vi "Rayon max.vi"(8 "error in (no error)":T1 caption="entrée d'erreur (pas d'erreur)", 10 "Capteur 3 ou 4":dbl[](array[numeric]), 11 "Capteur 2":dbl[](array[numeric])) -> (0 "error out":T1 caption="sortie d'erreur", 3 "Rayon max":dbl)   [LabVIEW 2018]
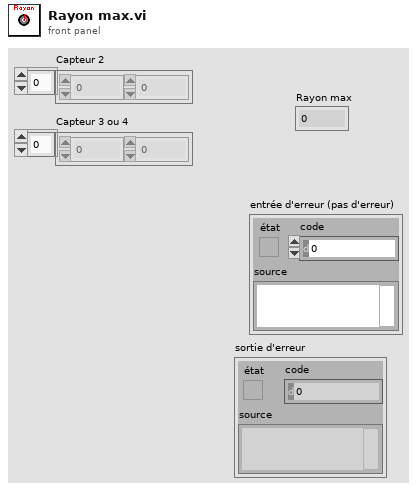
[diagram p1: front panel]
types:
  T1 = cluster{"état":bool, "code":i32, "source":string}
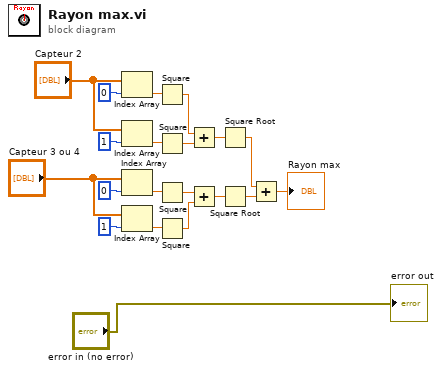
[diagram p0: block diagram]
diagram:
  n1 = Index Array(array="Capteur 2", index=0 ("indice")) -> (element=w16:dbl)
  n2 = Index Array(array="Capteur 2", index=1 ("indice")) -> (element=w17:dbl)
  n3 = Index Array(array="Capteur 3 ou 4", index=0 ("indice")) -> (element=w9:dbl)
  n4 = Index Array(array="Capteur 3 ou 4", index=1 ("indice")) -> (element=w10:dbl)
  n5 = Square(x=w16) -> (x^2=w14:dbl)
  n6 = Square(x=w17) -> (x^2=w15:dbl)
  n7 = Square(x=w9) -> (x^2=w7:dbl)
  n8 = Square(x=w10) -> (x^2=w8:dbl)
  n9 = Add(x=w14, y=w15) -> (x+y=w13:dbl)
  n10 = Add(x=w7, y=w8) -> (x+y=w6:dbl)
  n11 = Square Root(x=w13) -> (sqrt(x)=w4:dbl)
  n12 = Square Root(x=w6) -> (sqrt(x)=w3:dbl)
  n13 = Add(x=w4, y=w3) -> (x+y=→"Rayon max":dbl)
  "error out" <- "error in (no error)"
